vi "Trace Event Callback.vi"(4 "User Parameter":variant, 5 "Event Data":T1, 6 "Control Ref":refnum<k7>, 7 "Event Common Data":T2) -> ()   [LabVIEW 2015]
panel:
  out "error out":errorcluster
  out "ResultStatus":string
  out "Name":string
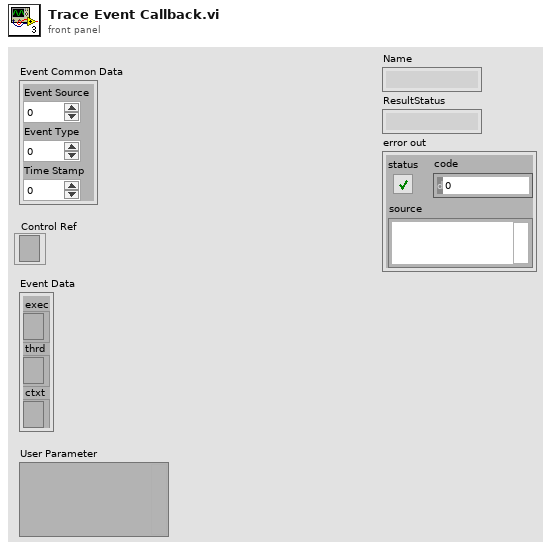
[diagram p1: front panel]
types:
  T1 = cluster{"exec":refnum<k7>, "thrd":refnum<k7>, "ctxt":refnum<k7>}
  T2 = cluster{"Event Source":i32, "Event Type":u32, "Time Stamp":u32}
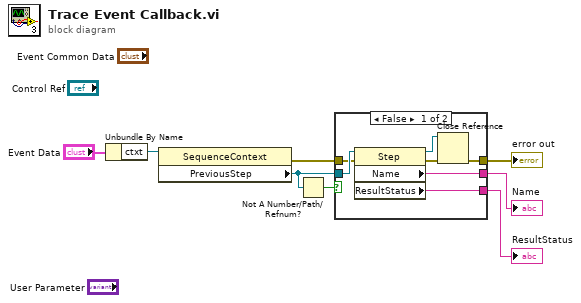
[diagram p0: block diagram]
diagram:
  n1 = Unbundle By Name("Event Data") -> ("ctxt"=w7:refnum<k7>)
  n2 = property class="SequenceContext"(reference=w7) -> (error out=w2:errorcluster, "PreviousStep"=w3:refnum<k7>)  [unwired: 1 in, 1 out]
  n3 = Not A Number/Path/Refnum?(number/path/refnum=w3) -> (NaN/Path/Refnum?=w4:bool)
  n4 = case shown="False" w4 {
    tunnel: [w13 _] -> w6
    tunnel: [w12 _] -> w5
    tunnel: w3 -> [w11 _]
    tunnel: w2 -> [w10 _]
    tunnel: [w9 _] -> w1
    frame False {
      n5 = property class="Step"(reference=w11, error in=w10) -> (reference out=w14:refnum<k7>, error out=w15:errorcluster, "Name"=w13:string, "ResultStatus"=w12:string)
      n6 = Close Reference(reference=w14, error in (no error)=w15) -> (error out=w9:errorcluster)
    }
    frame True {
    }
  }
  "Name" <- w6
  "ResultStatus" <- w5
  "error out" <- w1
